vi "Set gate delay step.vi"(8 "error in (no error)":errorcluster, 9 "t (0.000000)":dbl, 10 "Gate (A)":T1, 11 "VISA resource name":refnum<visa-resource-name>) -> (0 "error out":errorcluster, 3 "VISA resource name out":refnum<visa-resource-name>)   [LabVIEW 2009, in "SR400.lvlib"]
doc: "GY i { ,t }\nThe GY command sets and reads the gate delay\nscan step. i = 0 or 1 designates A gate or B gate\nand is required. If t is included, the selected gate\nscan step is set to t seconds where 0 <= t <=99.92E-3. The resolution is variable depending\nupon the 4 most significant digits of t.\n\n4 most significant digits -resolution in 4th digit\n\n1000 to 2048- 1 (1001,1002,1003,...)\n2048 to 4096 -2\n4096 to 8192 -4\n8192 to 9992 -8 (8192,8200,8208,...)\n\nFor example, near 10.00 ìs, the allowed values of\nt are 9.984 ìs, 9.992 ìs, 10.00 ìs, 10.01 ìs, etc.\nBelow 1.000 ìs, the resolution is 1 ns. Almost\nany value of t may be sent and the SR400 will\nround to the nearest allowed value. If t is absent,\nthe selected gate scan step is returned. The scan\nstep may be set and read even if the selected gate\nis not in the SCAN mode. Changing the scan step\nduring a scan will affect the gate position for the\nnext count period and all those that follow."
uses:
  SR400.lvlib
  Typedefs.llb/Gate.ctl
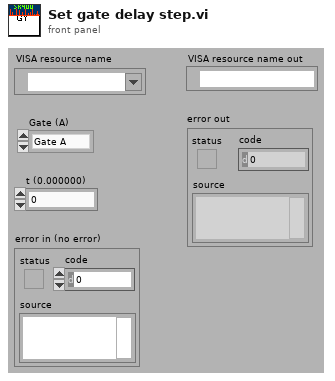
[diagram p1: front panel]
types:
  T1 = typedef "SR400.lvlib/Gate.ctl" = enum16{"Gate A", "Gate B"}
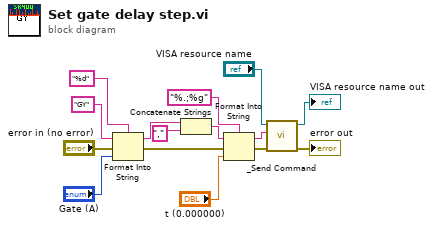
[diagram p0: block diagram]
diagram:
  n1 = Format Into String(format string="%d", initial string="GY" ("command"), error in="error in (no error)", "Gate (A)") -> (resulting string=w12:string, error out=w13:errorcluster)
  n2 = Concatenate Strings(w12, "," ("command")) -> (w7:string)
  n3 = Format Into String(format string="%.;%g", initial string=w7, error in=w13, "t (0.000000)") -> (resulting string=w4:string, error out=w3:errorcluster)
  n4 = call "_Send Command.vi"("error in (no error)"=w3, "Command"=w4, "VISA resource name"="VISA resource name") -> ("error out"=→"error out":errorcluster, "VISA resource name out"=→"VISA resource name out":refnum<visa-resource-name>)  [unwired: 1 in, 6 out]
